vi "Tabla estatus to UI.vi"(8 "error in (no error)":errorcluster, 10 "Tabla estatus":string[][](array[string]), 11 "Contabilidad in":refnum<class "Contabilidad.lvclass">) -> (0 "error out":errorcluster, 3 "Contabilidad out":refnum<class "Contabilidad.lvclass">)   [LabVIEW 2020, in "Contabilidad.lvlib" / "Contabilidad.lvclass"]
uses:
  Contabilidad.lvclass
  C:/Program Files (x86)/National Instruments/LabVIEW 2020/vi.lib/ActorFramework/Actor/Actor.lvclass
  Contabilidad.lvclass/Contabilidad.ctl
  <vilib>/ActorFramework/Actor/Actor.lvclass/Actor.ctl
  UI Messages/Obtain tabla estatus from Contabilidad Msg/Obtain tabla estatus from Contabilidad Msg.lvclass/Obtain tabla estatus from Contabilidad Msg.ctl
  <vilib>/ActorFramework/Message Enqueuer/Message Enqueuer.lvclass/Message Enqueuer.ctl
  <vilib>/ActorFramework/Message Enqueuer/Enqueue.vi
  UI Messages/Obtain tabla estatus from Contabilidad Msg/Obtain tabla estatus from Contabilidad Msg.lvclass
  C:/Program Files (x86)/National Instruments/LabVIEW 2020/vi.lib/ActorFramework/Message/Message.lvclass
  <vilib>/ActorFramework/Message Priority Queue/Priority Enqueue.vi
  <vilib>/ActorFramework/Actor/Actor.lvclass
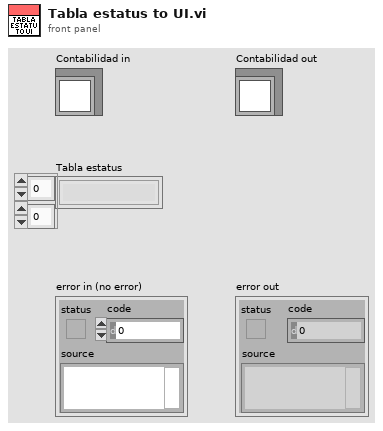
[diagram p1: front panel]
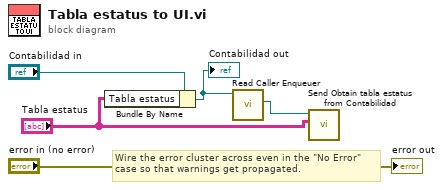
[diagram p0: block diagram]
diagram:
  # "Wire the error cluster across even in the \"No Error\"\ncase so that warnings get propagated."
  n1 = Bundle By Name(cluster="Contabilidad in", "Tabla estatus"="Tabla estatus") -> (w2:refnum<class "Contabilidad.lvclass">)
  "Contabilidad out" <- w2
  n2 = call <vilib>:"Read Caller Enqueuer.vi"("Actor"=w2) -> ("Caller Enqueuer"=w1:refnum<class "Message Enqueuer.lvclass">)  [unwired: 10 in]
  n3 = call "Send Obtain tabla estatus from Contabilidad.vi"("Tabla estatus"="Tabla estatus", "Message Enqueuer"=w1) -> ()  [unwired: 8 in, 2 out]
  "error out" <- "error in (no error)"
